vi "Do Preview.vi"(6 "Diagnostics Queue":refnum<queue>, 7 "Host Resources":T1, 8 "error in":errorcluster, 10 "Generated Data":string, 11 "Hardware Configuration in":T4) -> (0 "error out":errorcluster, 2 "Acquired Data":T13, 3 "Hardware Configuration out":T4)   [LabVIEW 2021, in "Load Frame.lvlib"]
doc: "Configure and read a single sample from the only channel in 'Hardware Configuration in'."
uses:
  Load Frame.lvlib
  Acquisition/Acquired Data.ctl
  Acquisition/Hardware Configuration.ctl
  Acquisition/Channel Settings.ctl
  Acquisition/IO Device.ctl
  Acquisition/Sensor Type.ctl
  Interval Timer/Repeat Interval.ctl
  Interval Timer/Interval Length.ctl
  Interval Timer/Interval Token.ctl
  Acquisition/IO Context.ctl
  Acquisition/IO API.ctl
  Acquisition/Host Resources.ctl
  Acquisition/Host Software Package.ctl
  Acquisition/Host IO Resource.ctl
  support/Message Queue/Message Cluster.ctl
  Acquisition/Acquisition.lvlib
  <resource>/objmgr/daqmx.rc
  Interval Timer/Interval Timer.lvlib
  support/Message Queue/Message Queue.lvlib
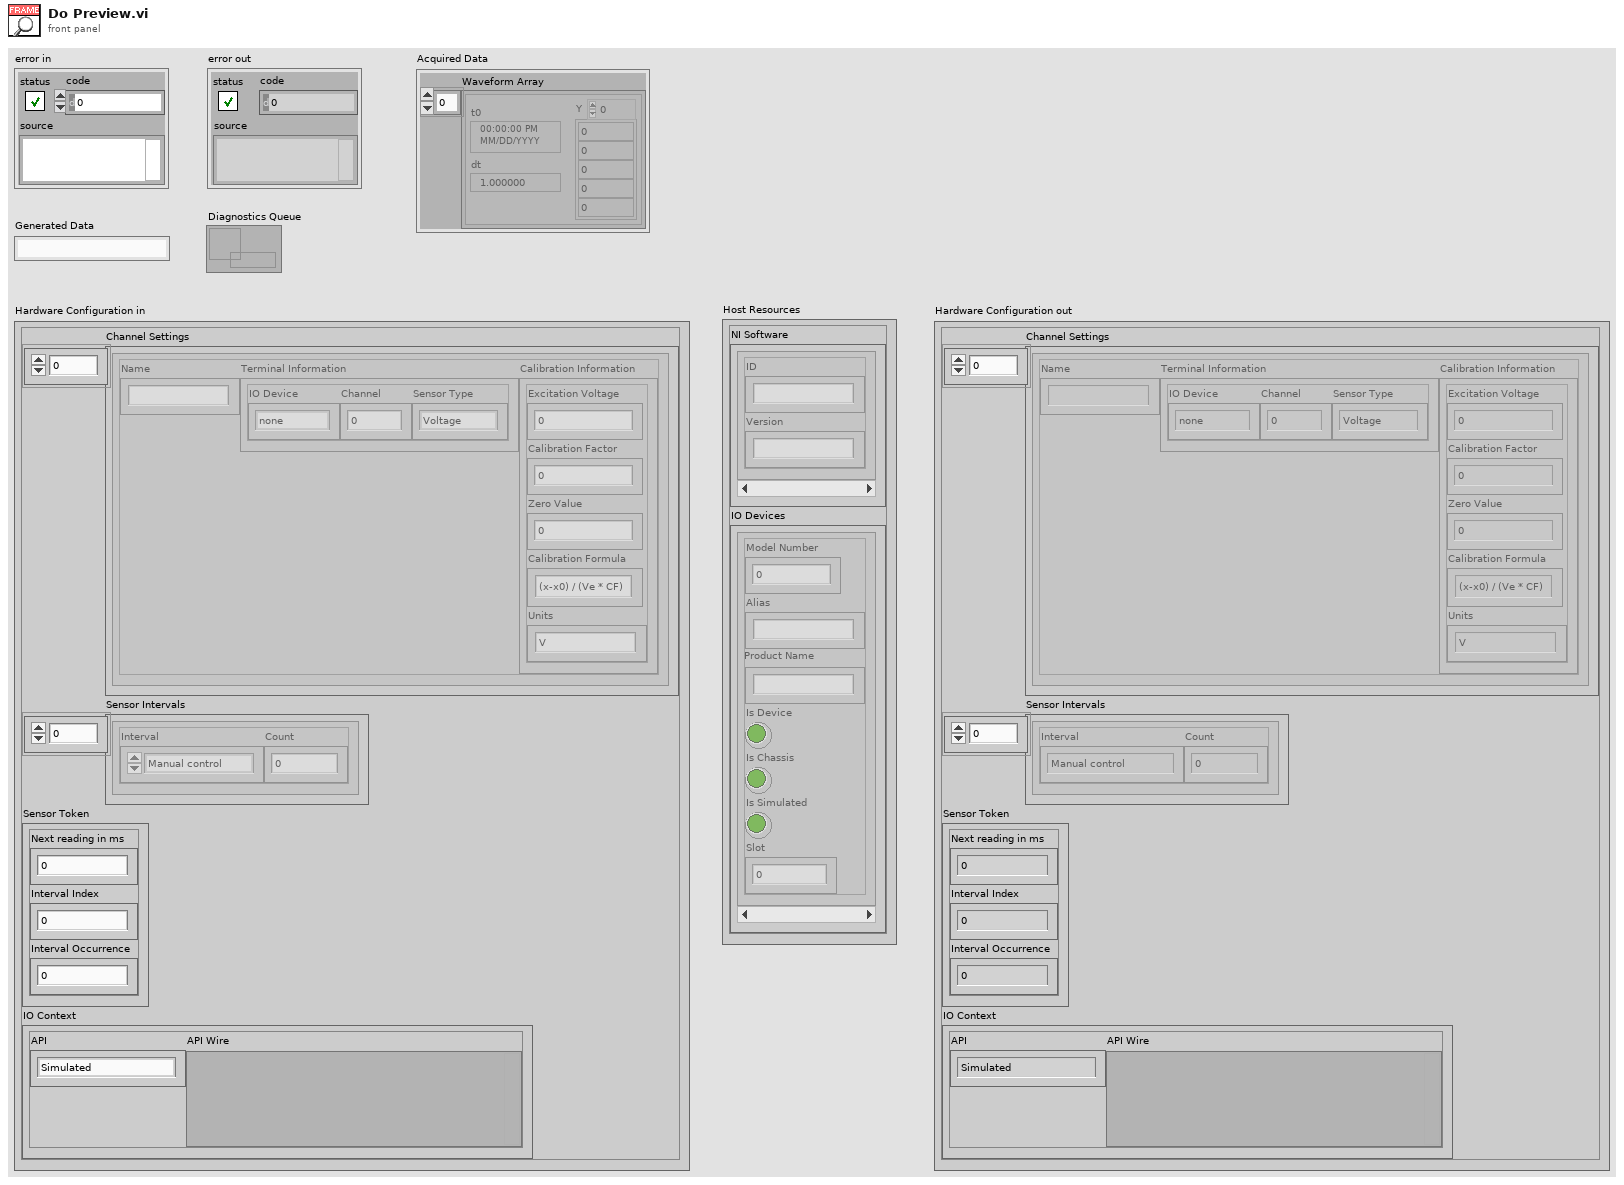
[diagram p1: front panel]
types:
  T1 = typedef "Acquisition.lvlib/Host Resources.ctl" = cluster{"NI Software":T2[], "IO Devices":T3[]}
  T2 = typedef "Acquisition.lvlib/Host Software Package.ctl" = cluster{"ID":string, "Version":string}
  T3 = typedef "Acquisition.lvlib/Host IO Resource.ctl" = cluster{"Model Number":u32, "Alias":string, "Product Name":string, "Is Device":bool, "Is Chassis":bool, "Is Simulated":bool, "Slot":i32}
  T4 = typedef "Acquisition.lvlib/Hardware Configuration.ctl" = cluster{"Channel Settings":T5[], "Sensor Intervals":T8[], "Sensor Token":T10, "IO Context":T11}
  T5 = typedef "Acquisition.lvlib/Channel Settings.ctl" = cluster{"Name":string, "Terminal Information":cluster{"IO Device":T6, "Channel":i32, "Sensor Type":T7}, "Calibration Information":cluster{"Excitation Voltage":dbl, "Calibration Factor":dbl, "Zero Value":dbl, "Calibration Formula":string, "Units":string}}
  T6 = typedef "Acquisition.lvlib/IO Device.ctl" = enum16{"none", "9219", "9401"}
  T7 = typedef "Acquisition.lvlib/Sensor Type.ctl" = enum16{"Voltage", "Load", "Pressure", "Encoder"}
  T8 = typedef "Interval Timer.lvlib/Repeat Interval.ctl" = cluster{"Interval":T9, "Count":i32}
  T9 = typedef "Interval Timer.lvlib/Interval Length.ctl" = enum16{"Manual control", "1 second", "10 seconds", "30 seconds", "60 seconds", "600 seconds", "1200 seconds", "3600 seconds"}
  T10 = typedef "Interval Timer.lvlib/Interval Token.ctl" = cluster{"Next reading in ms":u32, "Interval Index":i32, "Interval Occurrence":i32}
  T11 = typedef "Acquisition.lvlib/IO Context.ctl" = cluster{"API":T12, "API Wire":variant}
  T12 = typedef "Acquisition.lvlib/IO API.ctl" = enum16{"Simulated", "DAQmx"}
  T13 = typedef "Acquisition.lvlib/Acquired Data.ctl" = cluster{"Waveform Array":waveform(dbl)[]}
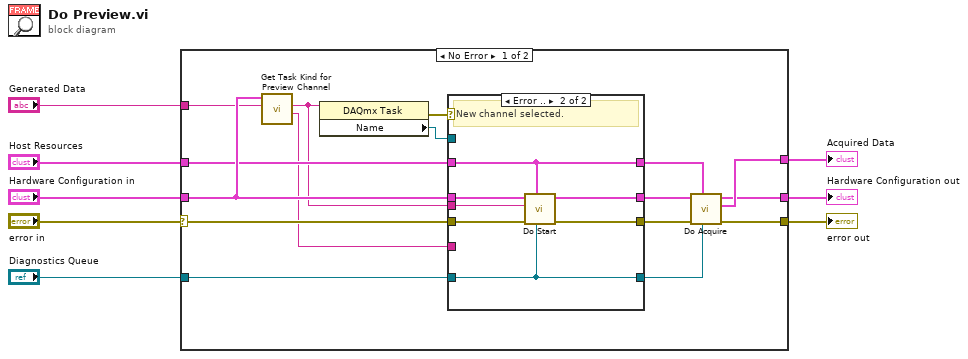
[diagram p0: block diagram]
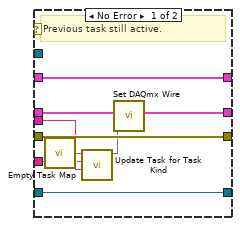
[diagram p2: hidden frame]
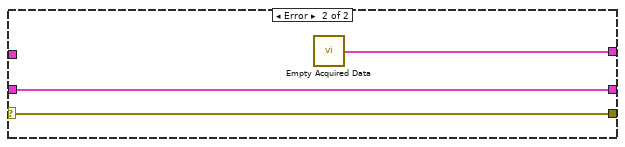
[diagram p3: hidden frame]
diagram:
  n1 = case shown="No Error" "error in" {
    selector: "error in" -> [w22 w43]
    tunnel: [w23 w43] -> w7
    tunnel: "Hardware Configuration in" -> [w15 w41]
    tunnel: [w24 w42] -> w5
    tunnel: "Generated Data" -> [w13 _]
    tunnel: [w19 w41] -> w4
    tunnel: "Host Resources" -> [w14 _]
    tunnel: "Diagnostics Queue" -> [w18 _]
    frame No Error {
      n2 = call "Get Task Kind for Preview Channel.vi"("Channel Index"=w13, "Hardware Configuration in"=w15) -> ("Task kind"=w12:string, "Task name"=w10:string)  [unwired: 8 in]
      n3 = property class="DAQmx Task"(reference=w10) -> (error out=w11:errorcluster, "Name"=w9:refnum<k21>)  [unwired: 1 in, 1 out]
      n4 = case shown="Error .." w11 {
        tunnel: w22 -> [w32 w36]
        tunnel: [w32 w40] -> w21
        tunnel: w15 -> [w33 w37]
        tunnel: [w31 w39] -> w20
        tunnel: w10 -> [w26 w38]
        tunnel: w14 -> [w30 w35]
        tunnel: w18 -> [w29 w34]
        tunnel: [w30 w35] -> w17
        tunnel: [w29 w34] -> w16
        tunnel: w12 -> [w25 _]
        tunnel: w9 -> [_ _]
        frame No Error {
          # "Previous task still active."
          n5 = call "Empty Task Map.vi"() -> ("Task Map"=w28:map{string, refnum<k21>})
          n6 = call "Update Task for Task Kind.vi"("DAQmx Task"=w26, "DAQmx Task prefix"=w25, "Task Map in"=w28) -> ("Task Map out"=w27:map{string, refnum<k21>})  [unwired: 8 in]
          n7 = call "Set DAQmx Wire.vi"("Task Map"=w27, "Hardware Configuration"=w33) -> ("Hardware Configuration out"=w31:T4)  [unwired: 7 in]
        }
        frame Error {
          # "New channel selected."
          n8 = call "Do Start.vi"("Diagnostics Queue"=w34, "Host Resources"=w35, "error in"=w36, "Generated Data"=w38, "Hardware Configuration in"=w37) -> ("error out"=w40:errorcluster, "Hardware Configuration out"=w39:T4)  [unwired: 4 in, 1 out]
        }
      }
      n9 = call "Do Acquire.vi"("Diagnostics Queue"=w16, "Host Resources"=w17, "error in"=w21, "Hardware Configuration in"=w20) -> ("error out"=w23:errorcluster, "Acquired Data"=w24:T13, "Hardware Configuration out"=w19:T4)  [unwired: 5 in]
    }
    frame Error {
      n10 = call "Empty Acquired Data.vi"() -> ("Empty Acquired Data"=w42:T13)
    }
  }
  "error out" <- w7
  "Acquired Data" <- w5
  "Hardware Configuration out" <- w4
